vi "color_alignment2.vi"(10 "NXT/EV3":T2, 11 "Begginning color":T1=enum."White") -> (0 "NXT/EV3 2":T2)   [LabVIEW 2016]
uses:
  parametros.ctl
  <vilib>/NXT/Block Support/NXT_InputPort.ctl
  <vilib>/NXT/Subs/LVHSConnector.ctl
  <vilib>/NXT/LegoClasses/BrickReference/BrickReference.lvclass
  <vilib>/NXT/Subs/ColorSensorColors.ctl
  <vilib>/NXT/Block Support/NXT_OutputPort.ctl
  <vilib>/NXT/NXTIO Xnodes/NXTIONodeSubVIs/NXTMoveMotors.vi
  <vilib>/NXT/NXTIO Xnodes/AddressXNode/NXTIOAddress.xnode
  <vilib>/NXT/NXTIO Xnodes/NXTIOXNode/NXTIO.xnode
panel:
  out "Collor":T1
  in  "Parâmetros Iniciais":T3={"Gyro Port"=0, "Sensor - Left"=3, "Sensor - Right"=2, "     Color \nSensor Port"=1, "Kp Front"=0.5, "Motor speed"=-15, "Distance to street"=15.0, "Motor speed turns"=16, "Kp Curvas"=0.3} {"Kp Front" format="%.3f"; "Color \nSensor Port" items=["Port 1", "Port 2", "Port 3", "Port 4"]; "Sensor - Right" items=["Port 1", "Port 2", "Port 3", "Port 4"]; "Sensor - Left" items=["Port 1", "Port 2", "Port 3", "Port 4"]; "Gyro Port" items=["Port 1", "Port 2", "Port 3", "Port 4"]}
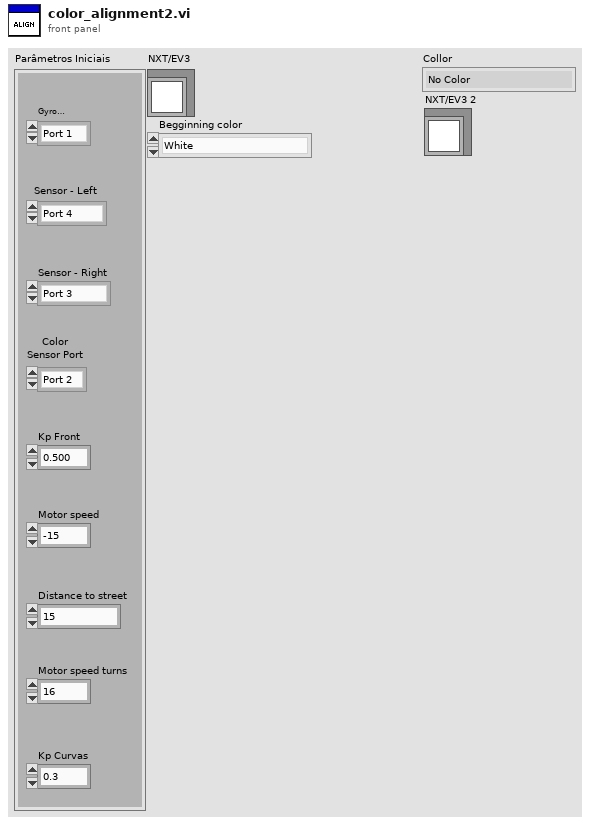
[diagram p1: front panel]
types:
  T1 = typedef "ColorSensorColors.ctl" = enum16{"No Color", "Black", "Blue", "Green", "Yellow", "Red", "White", "Brown"}
  T2 = typedef "LVHSConnector.ctl" = refnum<class "BrickReference.lvclass">
  T3 = typedef "parametros.ctl" = cluster{"Gyro Port":T4, "Sensor - Left":T4, "Sensor - Right":T4, "     Color \nSensor Port":T4, "Kp Front":dbl, "Motor speed":i32, "Distance to street":dbl, "Motor speed turns":i32, "Kp Curvas":dbl}
  T4 = typedef "NXT_InputPort.ctl" = u32
  T5 = typedef "NXT_OutputPort.ctl" = u8
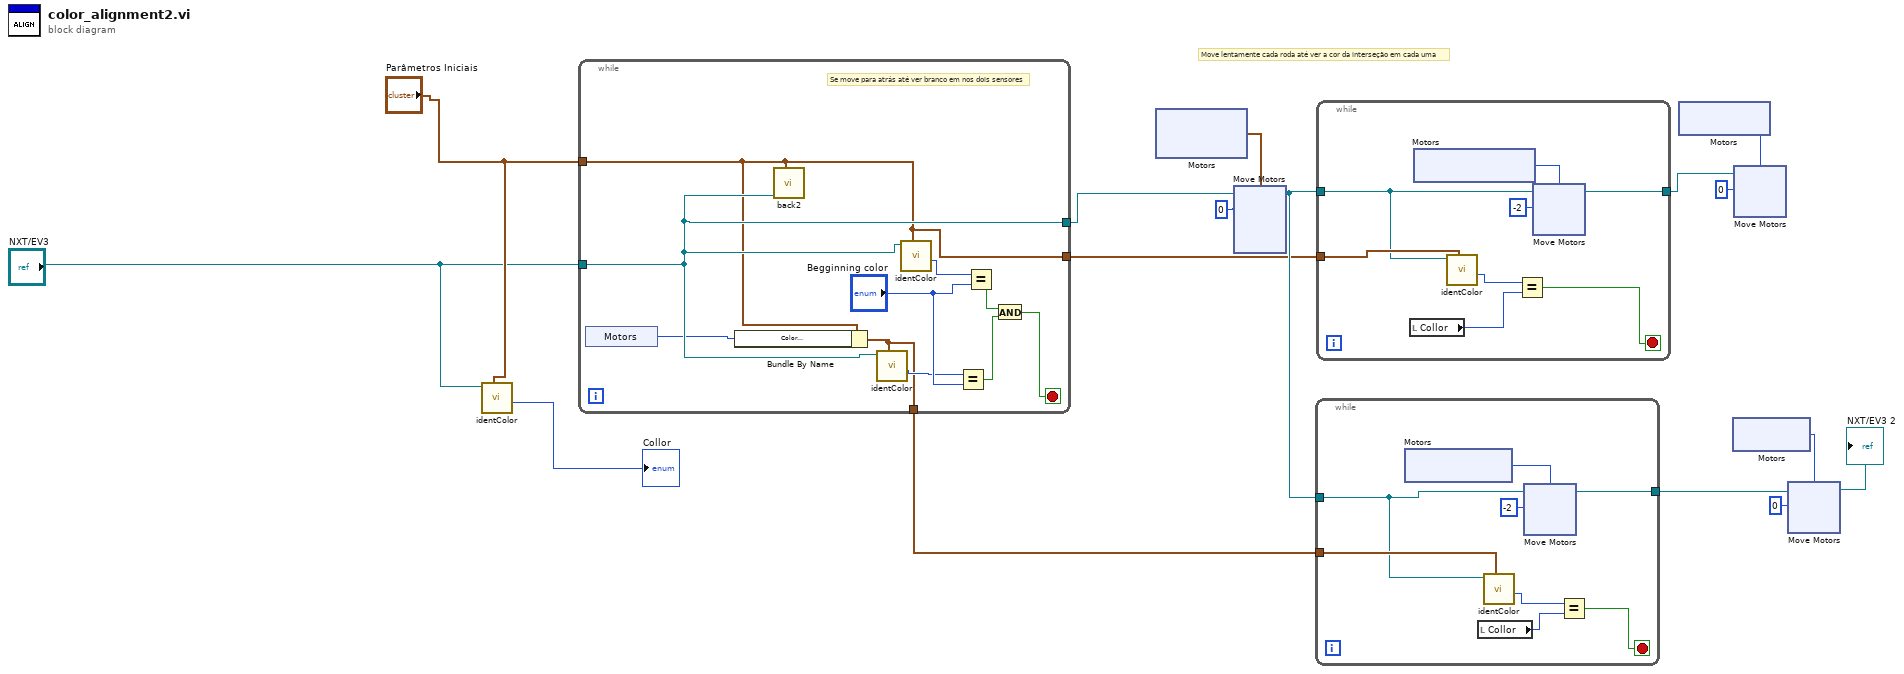
[diagram p0: block diagram]
diagram:
  w1 = i8 0 ("Power/Speed 1")
  # "Move lentamente cada roda até ver a cor da interseção em cada uma"
  n1 = call "identColor.vi"("Parâmetros Ini"="Parâmetros Iniciais", "NXT/EV3"="NXT/EV3") -> ("Collor"=→"Collor":T1)  [unwired: 8 in, 1 out]
  n2 = while {
    tunnel: "NXT/EV3" -> [w21]
    tunnel: "Parâmetros Iniciais" -> [w18]
    tunnel: [w21] -> w13
    tunnel: [w18] -> w5
    tunnel: [w17] -> w4
    stop <- w24 stop-if-true
    # "Se move para atrás até ver branco em nos dois sensores"
    n3 = xnode "Motors"() -> ("Sensor"=w19:T4)
    n4 = Bundle By Name(cluster=w18, "Color \nSensor Port"=w19) -> (w17:T3)
    n5 = call "back2.vi"("Parâmetros Ini 2"=w18, "NXT/EV3"=w21) -> ()  [unwired: 9 in, 1 out]
    n6 = call "identColor.vi"("Parâmetros Ini"=w17, "NXT/EV3"=w21) -> ("Collor"=w20:T1)  [unwired: 8 in, 1 out]
    n7 = call "identColor.vi"("Parâmetros Ini"=w18, "NXT/EV3"=w21) -> ("Collor"=w22:T1)  [unwired: 8 in, 1 out]
    n8 = Equal?(x=w20, y="Begginning color") -> (x = y?=w25:bool)
    n9 = Equal?(x=w22, y="Begginning color") -> (x = y?=w26:bool)
    n10 = And(x=w26, y=w25) -> (x .and. y?=w24:bool)
  }
  n11 = xnode "Motors"() -> ("Motor"=w14:cluster{"Port":T5, "Port":T5})
  n12 = xnode "Move Motors"("Power/Speed 2"=w1, "Power/Speed 1"=w1, "Motors"=w14, "NXT/EV3"=w13) -> ("NXT/EV3"=w8:T2)
  n13 = while {
    tunnel: w8 -> [w28]
    tunnel: [w31] -> w10
    tunnel: w4 -> [w30]
    stop <- w32 stop-if-true
    n14 = xnode "Motors"() -> ("Motor"=w35:T5)
    n15 = local read "Collor"() -> (w33:T1)
    n16 = call "identColor.vi"("Parâmetros Ini"=w30, "NXT/EV3"=w28) -> ("Collor"=w29:T1)  [unwired: 8 in, 1 out]
    n17 = xnode "Move Motors"("Power/Speed 1"=i8 -2, "Motors"=w35, "NXT/EV3"=w28) -> ("NXT/EV3"=w31:T2)
    n18 = Equal?(x=w29, y=w33) -> (x = y?=w32:bool)
  }
  n19 = while {
    tunnel: w8 -> [w45]
    tunnel: [w49] -> w9
    tunnel: w5 -> [w46]
    stop <- w47 stop-if-true
    n20 = local read "Collor"() -> (w48:T1)
    n21 = xnode "Motors"() -> ("Motor"=w51:T5)
    n22 = call "identColor.vi"("Parâmetros Ini"=w46, "NXT/EV3"=w45) -> ("Collor"=w44:T1)  [unwired: 8 in, 1 out]
    n23 = Equal?(x=w44, y=w48) -> (x = y?=w47:bool)
    n24 = xnode "Move Motors"("Power/Speed 1"=i8 -2, "Motors"=w51, "NXT/EV3"=w45) -> ("NXT/EV3"=w49:T2)
  }
  n25 = xnode "Motors"() -> ("Motor"=w12:T5)
  n26 = xnode "Motors"() -> ("Motor"=w11:T5)
  n27 = xnode "Move Motors"("Power/Speed 1"=i8 0, "Motors"=w12, "NXT/EV3"=w9) -> ()  [unwired: 1 out]
  n28 = xnode "Move Motors"("Power/Speed 1"=i8 0, "Motors"=w11, "NXT/EV3"=w10) -> ("NXT/EV3"=→"NXT/EV3 2":T2)
